vi "TEST_3DOF.vi"() -> ()   [LabVIEW 2013]
uses:
  <vilib>/Instr/_visa.llb/VISA Configure Serial Port (Instr).vi
panel:
  out "바이트":u32
  in  "콤보 박스":string(combo)
  in  "정지":bool
  in  "VISA 리소스 이름":refnum<visa-resource-name>="COM3"
  in  "통신속도":u32=9600
  out "문자열":string
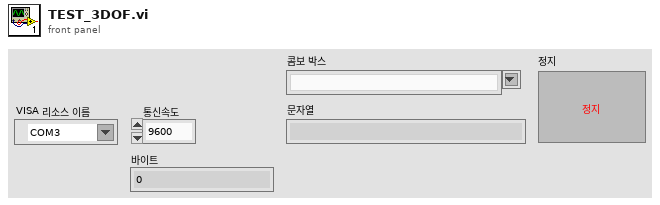
[diagram p1: front panel]
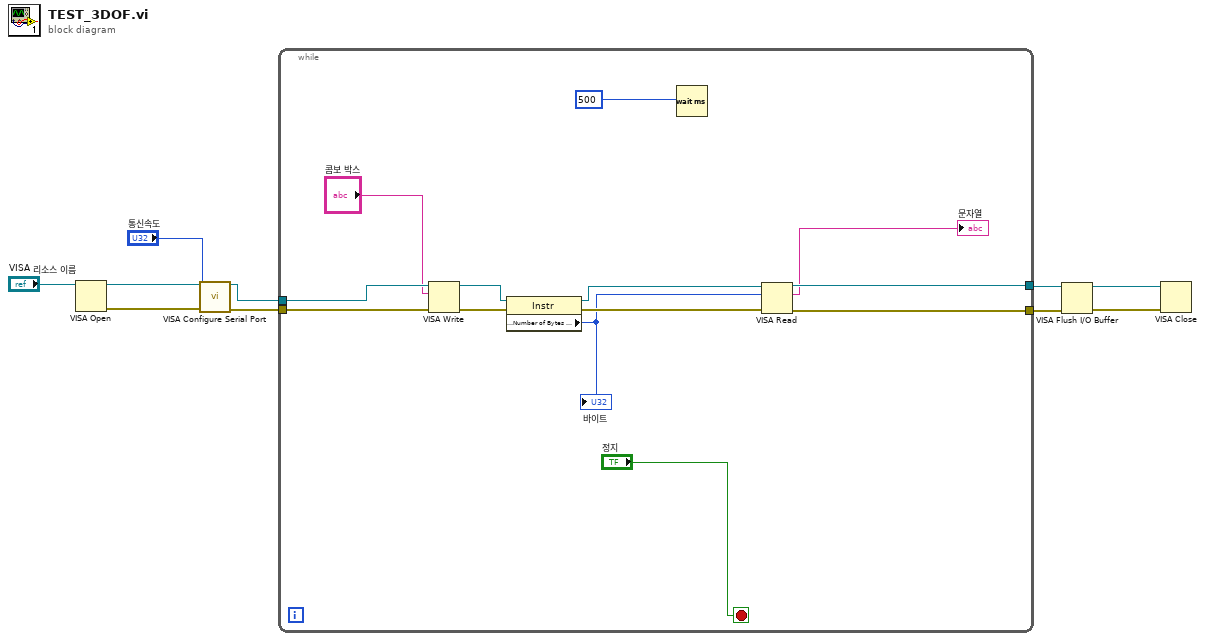
[diagram p0: block diagram]
diagram:
  n1 = VISA Open(VISA resource name="VISA 리소스 이름") -> (VISA resource name=w10:refnum<visa-resource-name>, error out=w9:errorcluster)  [unwired: 4 in]
  n2 = call-poly "VISA Configure Serial Port"("VISA resource name"=w10, "baud rate (9600)"="통신속도", "error in (no error)"=w9) -> ("VISA resource name out"=w6:refnum<visa-resource-name>, "error out"=w7:errorcluster)  [unwired: 11 in]
  n3 = while {
    tunnel: w7 -> [w20]
    tunnel: w6 -> [w19]
    tunnel: [w22] -> w4
    tunnel: [w21] -> w3
    stop <- "정지" stop-if-true
    n4 = VISA Write(VISA resource name=w19, write buffer="콤보 박스", error in (no error)=w20) -> (VISA resource name out=w14:refnum<visa-resource-name>, error out=w17:errorcluster)  [unwired: 1 out]
    n5 = property class="Instr"(reference=w14, error in=w17) -> (reference out=w15:refnum<visa-resource-name>, error out=w16:errorcluster, "Serial Settings:Number of Bytes at Serial Port"=w13:u32)
    "바이트" <- w13
    n6 = Wait (ms)(milliseconds to wait=u32 500 ("대기 시간(ms)")) -> ()  [unwired: 1 out]
    n7 = VISA Read(VISA resource name=w15, byte count=w13, error in (no error)=w16) -> (VISA resource name out=w21:refnum<visa-resource-name>, read buffer=→"문자열":string, error out=w22:errorcluster)  [unwired: 1 out]
  }
  n8 = VISA Flush I/O Buffer(VISA resource name=w3, error in (no error)=w4) -> (VISA resource name out=w2:refnum<visa-resource-name>, error out=w1:errorcluster)  [unwired: 1 in]
  n9 = VISA Close(VISA resource name=w2, error in (no error)=w1) -> ()  [unwired: 1 out]
